vi "Send Query 9620.vi"(8 "error in (no error)":errorcluster, 10 "Query":string, 11 "VISA resource name":refnum<visa-resource-name>="COM3") -> (0 "error out":errorcluster, 2 "read buffer":string, 3 "VISA resource name out":refnum<visa-resource-name>)   [LabVIEW 2017]
panel:
  out "how many times it had to read":i32
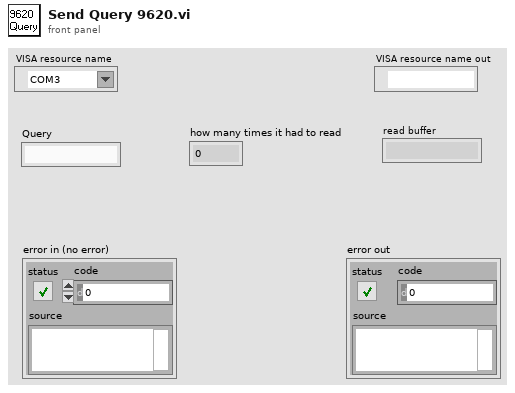
[diagram p1: front panel]
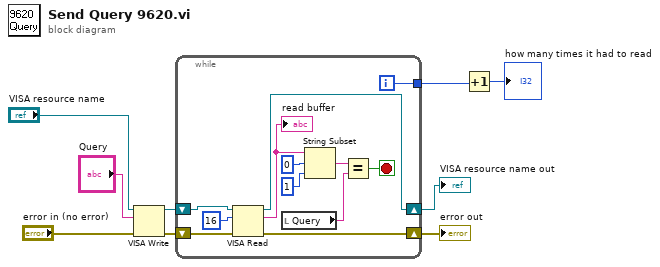
[diagram p0: block diagram]
diagram:
  n1 = VISA Write(VISA resource name="VISA resource name", write buffer="Query", error in (no error)="error in (no error)") -> (VISA resource name out=w7:refnum<visa-resource-name>, error out=w6:errorcluster)  [unwired: 1 out]
  n2 = while {
    shift-right: [w20] -> w8
    shift-left: w7 -> [w19]
    shift-right: [w21] -> w9
    shift-left: w6 -> [w18]
    tunnel: [w10] -> w2
    i -> [w10]
    stop <- w11 stop-if-true
    n3 = VISA Read(VISA resource name=w19, byte count=u32 16, error in (no error)=w18) -> (VISA resource name out=w20:refnum<visa-resource-name>, read buffer=w16:string, error out=w21:errorcluster)  [unwired: 1 out]
    "read buffer" <- w16
    n4 = local read "Query"() -> (w12:string)
    n5 = String Subset(string=w16, offset (0)=0, length (rest)=1 ("length (rest)")) -> (substring=w13:string)
    n6 = Equal?(x=w13, y=w12) -> (x = y?=w11:bool)
  }
  "VISA resource name out" <- w8
  "error out" <- w9
  n7 = Increment(x=w2) -> (x+1=→"how many times it had to read":i32)
